vi "telnet_com.vi"(0 "HIFU ip":string="192.168.1.20") -> ()   [LabVIEW 2016]
uses:
  <vilib>/addons/internet/NI_InternetTK_Core_VIs.lvlib
panel:
  in  "port":u32=23
  in  "stop":bool
  in  "log":string
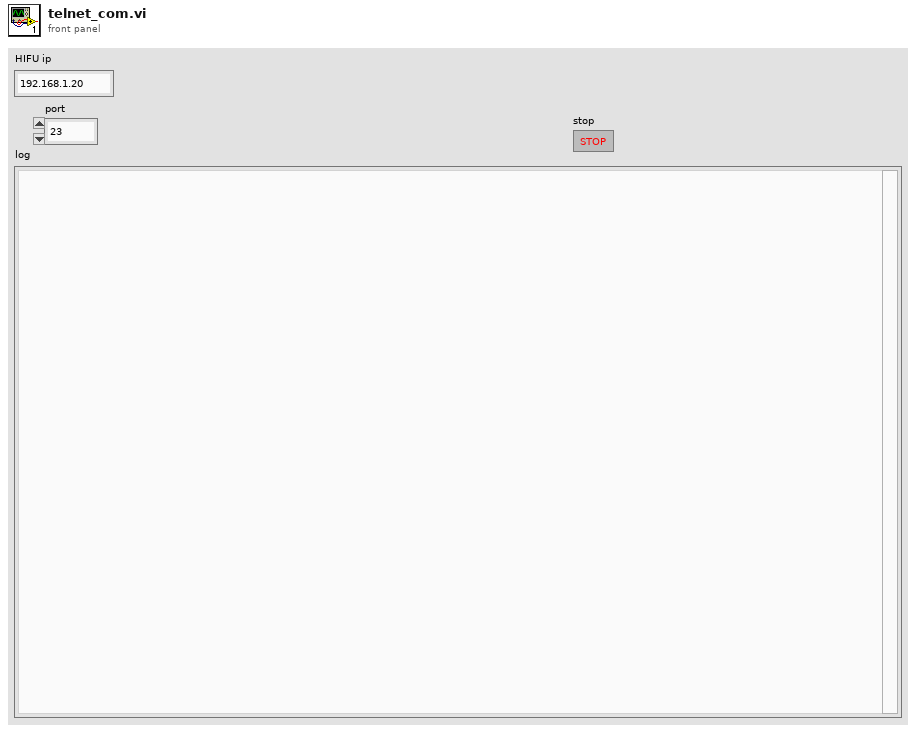
[diagram p1: front panel]
types:
  T1 = typedef "Telnet Session.ctl" = refnum<k1>
  T2 = typedef "eventvkey.ctl" = enum16{"ASCII", "Enter", "Return", "Shift", "Ctrl", "Alt", "Cmd", "Opt", "Caps", "NumLock", "Clear", "Break", "Up", "Down", "Left", "Right", "Insert", "Delete", "Home", "End", "PageUp", "PageDown", "Escape", "Help", "Pause", "ScrollLock", "F1", "F2", "F3", "F4", "F5", "F6", "F7", "F8", "F9", "F10", "F11", "F12", "F13", "F14", "F15", "F16", "F17", "F18", "F19", "F20", "F21", "F22", "F23", "F24", "Play", "VolumeUp", "VolumeDown", "Mute", "Two Byte Char"}
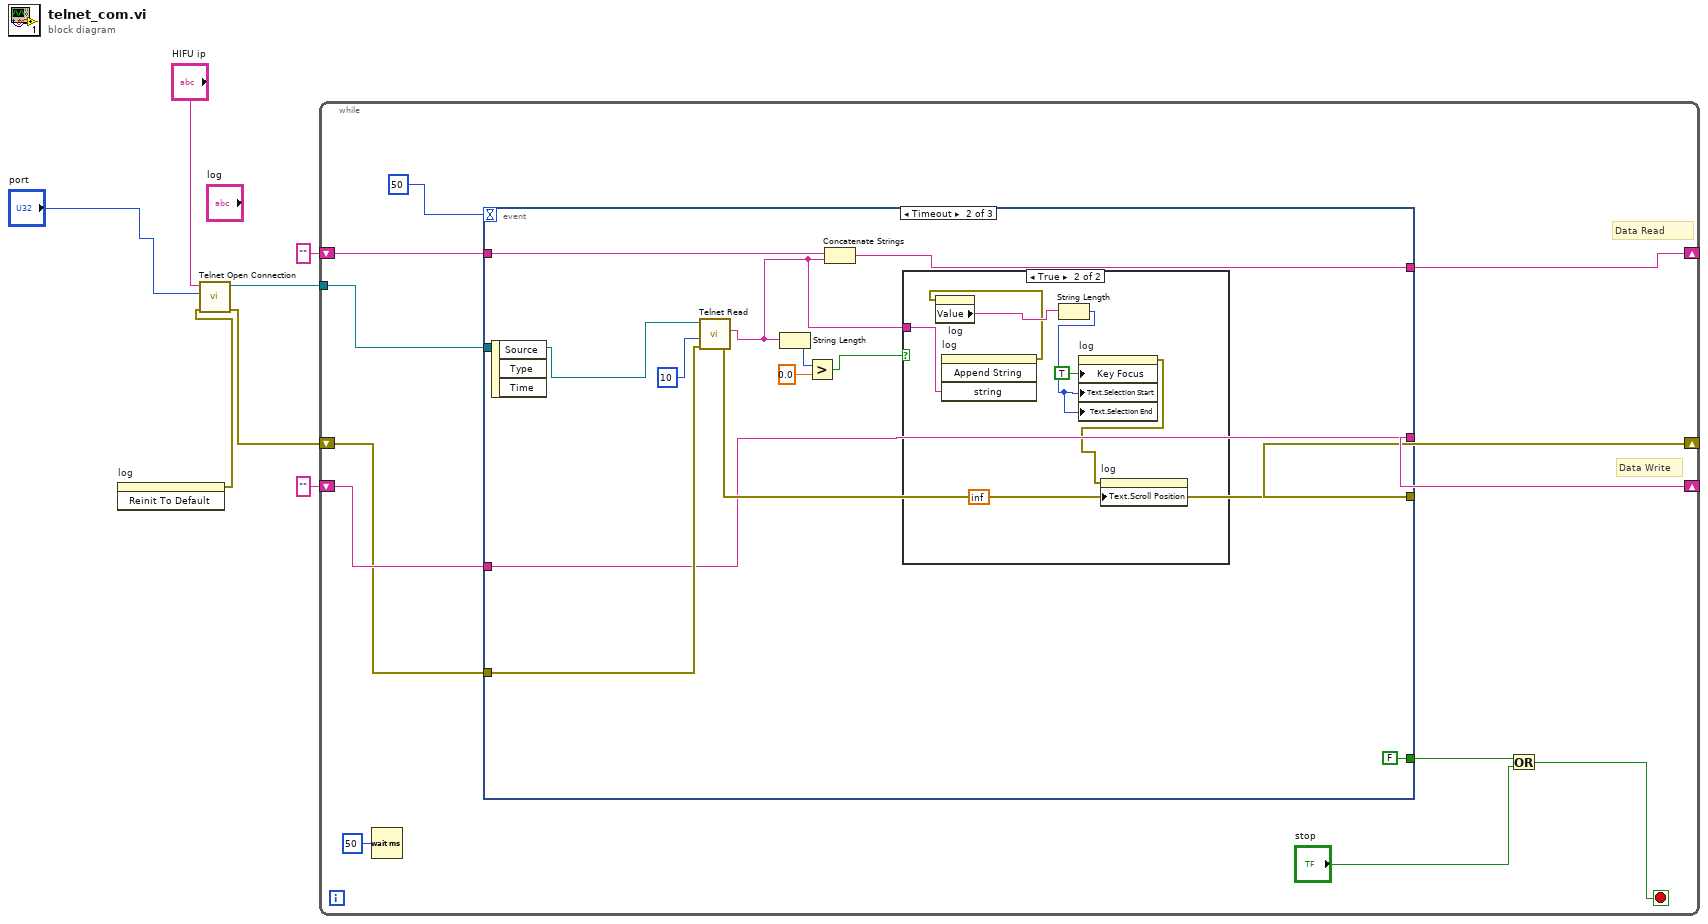
[diagram p0: block diagram]
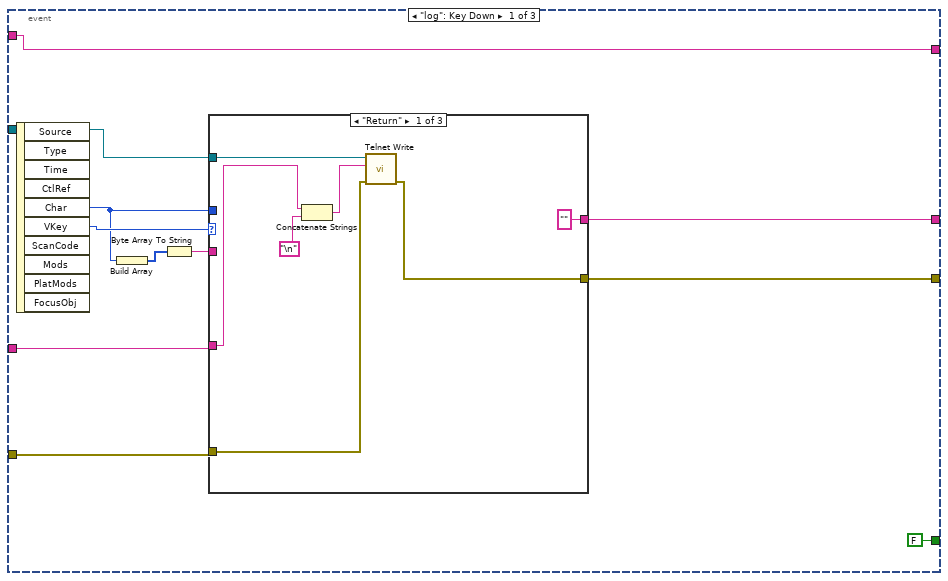
[diagram p2: hidden frame]
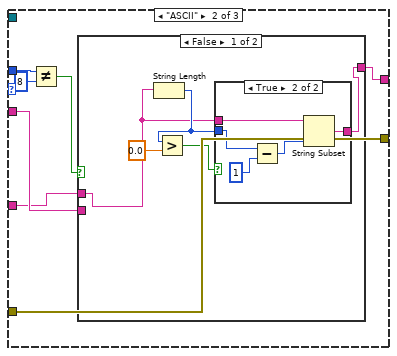
[diagram p3: hidden frame]
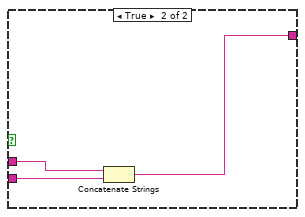
[diagram p5: hidden frame]
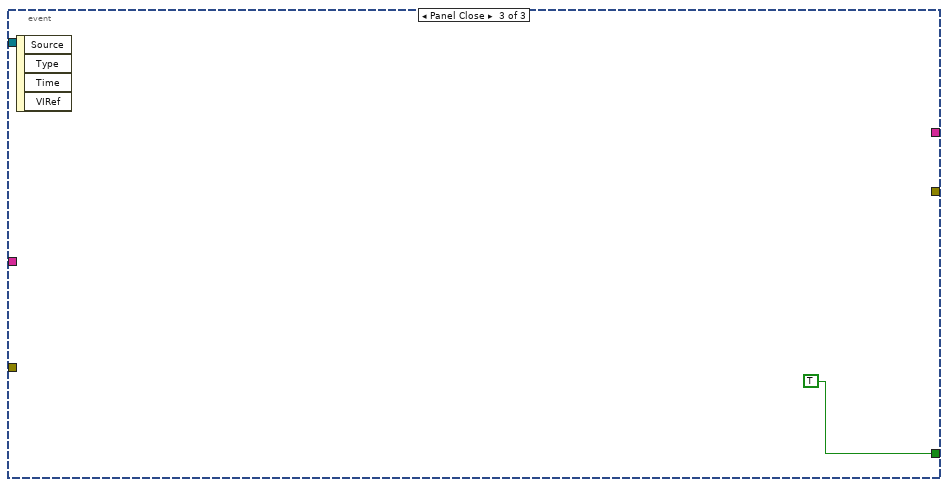
[diagram p8: hidden frame]
diagram:
  n1 = invoke on="log" class="Str" method="Reinit To Default"() -> (error out=w4:errorcluster)  [unwired: 3 in, 2 out]
  n2 = call <vilib>:"Telnet Open Connection.vi"("error in (no error)"=w4, "remote port (23)"="port", "address"="HIFU ip") -> ("error out"=w6:errorcluster, "telnet connection"=w7:T1)  [unwired: 7 in]
  n3 = while {
    tunnel: w7 -> [w15]
    shift-right: [w11] -> _
    shift-left: "" -> [w12]
    shift-right: [w17] -> _
    shift-left: "" -> [w18]
    shift-right: [w13] -> _
    shift-left: w6 -> [w16]
    stop <- w9 stop-if-true
    # "Data Write"
    # "Data Read"
    n4 = Wait (ms)(milliseconds to wait=u32 50) -> ()  [unwired: 1 out]
    n5 = event shown="[1] Timeout" {
      selector: _ -> [_ _ _]
      dyn-events: _ -> [_ _ _]
      timeout: 50 -> [_ _ _]
      tunnel: w15 -> [w30 w72 _]
      tunnel: [w26 w66 _] -> w17
      tunnel: w18 -> [w25 w66 _]
      tunnel: w16 -> [w24 w70 _]
      tunnel: [w23 w69 _] -> w13
      tunnel: w12 -> [w21 w68 _]
      tunnel: [w21 w67 _] -> w11
      tunnel: [FALSE FALSE TRUE] -> w8
      event "log": Key Down {
        n6 = event-data() -> ("Char"=w22:i16, "VKey"=w29:T2)  [unwired: 1 in, 8 out]
        n7 = Build Array(w22) -> (w28:i16[])
        n8 = Byte Array To String(unsigned byte array=w28) -> (string=w27:string)
        n9 = case shown="\"Return\"" w29 {
          tunnel: w30 -> [w37 _ _]
          tunnel: w27 -> [_ w44 _]
          tunnel: ["" w43 w60] -> w26
          tunnel: w25 -> [w32 w42 w60]
          tunnel: w24 -> [w35 w41 w59]
          tunnel: [w34 w41 w59] -> w23
          tunnel: w22 -> [_ w40 _]
          frame "Return" {
            n10 = Concatenate Strings(w32, "\n") -> (w31:string)
            n11 = call <vilib>:"Telnet Write.vi"("error in (no error)"=w35, "data in"=w31, "telnet connection"=w37) -> ("error out"=w34:errorcluster)  [unwired: 4 in, 2 out]
          }
          frame "ASCII" {
            n12 = Not Equal?(x=w40, y=i16 8) -> (x != y?=w38:bool)
            n13 = case shown="False" w38 {
              tunnel: w44 -> [_ w58]
              tunnel: [w45 w57] -> w43
              tunnel: w42 -> [w46 w56]
              frame False {
                n14 = String Length(string=w46) -> (length=w47:i32)
                n15 = Greater?(x=w47, y=0.0) -> (0:w48:bool)
                n16 = case shown="True" w48 {
                  tunnel: w46 -> [w50 w55]
                  tunnel: w47 -> [_ w54]
                  tunnel: [w50 w51] -> w45
                  frame False {
                  }
                  frame True {
                    n17 = Subtract(x=w54, y=1) -> (x-y=w52:i32)
                    n18 = String Subset(string=w55, length (rest)=w52) -> (substring=w51:string)  [unwired: 1 in]
                  }
                }
              }
              frame True {
                n19 = Concatenate Strings(w56, w58) -> (w57:string)
              }
            }
          }
          frame "Shift", Default {
          }
        }
      }
      event Timeout {
        n20 = event-data() -> ()  [unwired: 1 in, 3 out]
        n21 = call <vilib>:"Telnet Read.vi"("error in (no error)"=w70, "timeout ms (25000)"=10, "telnet connection"=w72) -> ("error out"=w69:errorcluster, "data out"=w62:string)  [unwired: 4 in, 1 out]
        n22 = String Length(string=w62) -> (length=w64:i32)
        n23 = Greater?(x=w64, y=0.0) -> (0:w63:bool)
        n24 = Concatenate Strings(w68, w62) -> (w67:string)
        n25 = case shown="True" w63 {
          tunnel: w62 -> [_ w79]
          frame False {
          }
          frame True {
            n26 = invoke on="log" class="Str" method="Append String"("string"=w79) -> (error out=w75:errorcluster)  [unwired: 3 in, 3 out]
            n27 = property on="log" class="Str"(error in=w75) -> ("Value"=w78:string)  [unwired: 1 in, 2 out]
            n28 = String Length(string=w78) -> (length=w77:i32)
            n29 = property on="log" class="Str"("Key Focus"=TRUE, "Text.Selection Start"=w77, "Text.Selection End"=w77) -> (error out=w73:errorcluster)  [unwired: 2 in, 1 out]
            n30 = property on="log" class="Str"(error in=w73, "Text.Scroll Position"=inf) -> ()  [unwired: 1 in, 2 out]
          }
        }
      }
      event Panel Close {
        n31 = event-data() -> ()  [unwired: 1 in, 4 out]
      }
    }
    n32 = Or(x=w8, y="stop") -> (x .or. y?=w9:bool)
  }
